vi "Signal2.vi"(10 "Iteration":i32) -> (0 "Stop Loop":bool, 2 "Output":dbl)   [LabVIEW 2019]
panel:
  in  "Loop":i32
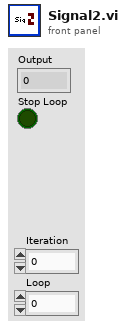
[diagram p1: front panel]
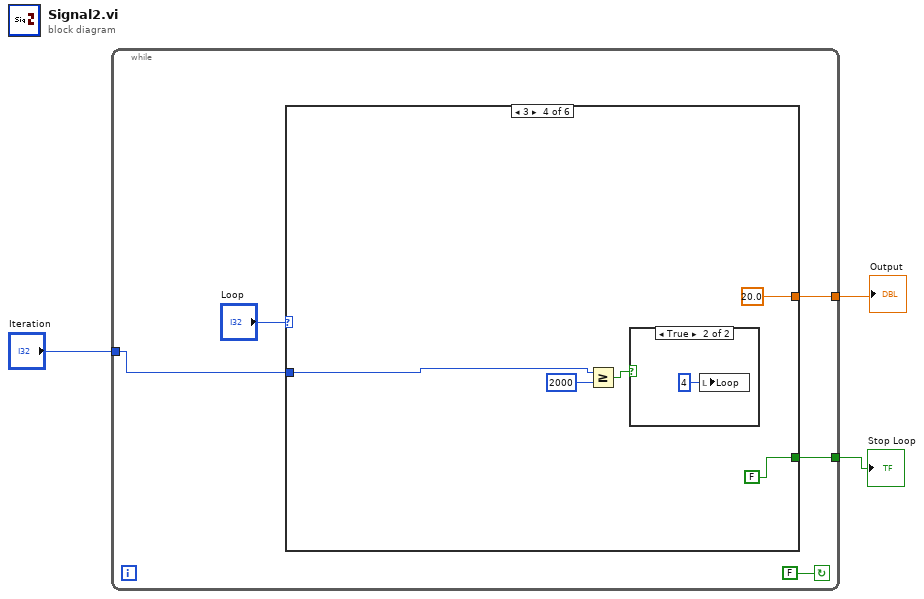
[diagram p0: block diagram]
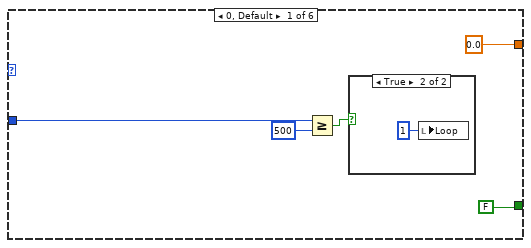
[diagram p2: hidden frame]
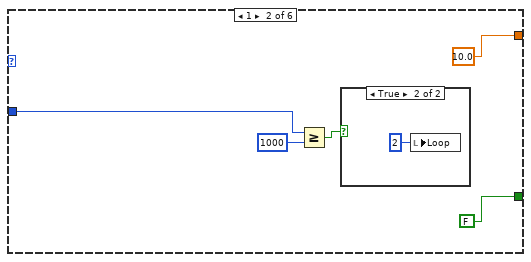
[diagram p4: hidden frame]
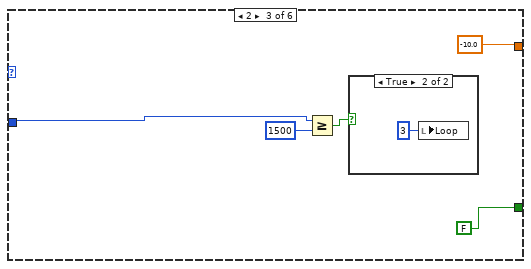
[diagram p6: hidden frame]
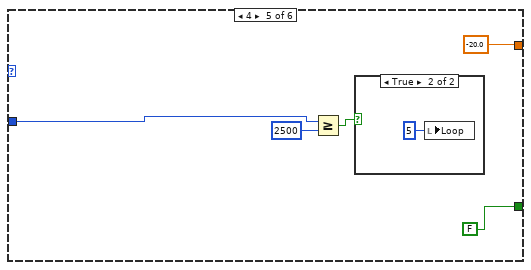
[diagram p9: hidden frame]
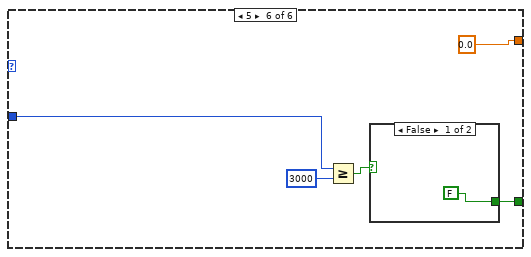
[diagram p11: hidden frame]
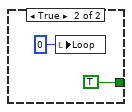
[diagram p12: hidden frame]
diagram:
  n1 = while {
    tunnel: "Iteration" -> [w6]
    tunnel: [w5] -> w2
    tunnel: [w4] -> w1
    stop <- FALSE continue-if-true
    n2 = case shown="3" "Loop" {
      tunnel: w6 -> [w13 w16 w22 w28 w34 w40]
      tunnel: [0.0 ("Output") 10.0 ("Output") -10.0 ("Output") 20.0 ("Output") -20.0 ("Output") 0.0 ("Output")] -> w5
      tunnel: [FALSE FALSE FALSE FALSE FALSE w39] -> w4
      frame 0, Default {
        n3 = Greater Or Equal?(x=w13, y=500) -> (x >= y?=w10:bool)
        n4 = case shown="True" w10 {
          frame False {
          }
          frame True {
            n5 = local write "Loop"(1 ("Loop")) -> ()
          }
        }
      }
      frame 1 {
        n6 = Greater Or Equal?(x=w16, y=1000) -> (x >= y?=w19:bool)
        n7 = case shown="True" w19 {
          frame False {
          }
          frame True {
            n8 = local write "Loop"(2 ("Loop")) -> ()
          }
        }
      }
      frame 2 {
        n9 = Greater Or Equal?(x=w22, y=1500) -> (x >= y?=w25:bool)
        n10 = case shown="True" w25 {
          frame False {
          }
          frame True {
            n11 = local write "Loop"(3 ("Loop")) -> ()
          }
        }
      }
      frame 3 {
        n12 = Greater Or Equal?(x=w28, y=2000) -> (x >= y?=w31:bool)
        n13 = case shown="True" w31 {
          frame False {
          }
          frame True {
            n14 = local write "Loop"(4 ("Loop")) -> ()
          }
        }
      }
      frame 4 {
        n15 = Greater Or Equal?(x=w34, y=2500) -> (x >= y?=w37:bool)
        n16 = case shown="True" w37 {
          frame False {
          }
          frame True {
            n17 = local write "Loop"(5 ("Loop")) -> ()
          }
        }
      }
      frame 5 {
        n18 = Greater Or Equal?(x=w40, y=3000) -> (x >= y?=w43:bool)
        n19 = case shown="False" w43 {
          tunnel: [FALSE ("Stop Loop") TRUE ("Stop Loop")] -> w39
          frame False {
          }
          frame True {
            n20 = local write "Loop"(0 ("Loop")) -> ()
          }
        }
      }
    }
  }
  "Output" <- w2
  "Stop Loop" <- w1
